vi "Basic Call Object Method.vi"(8 "Error In":errorcluster, 9 "args":string, 10 "method":string, 11 "object name":string) -> (0 "Error Out":errorcluster, 3 "concatened string":string)   [LabVIEW 2014]
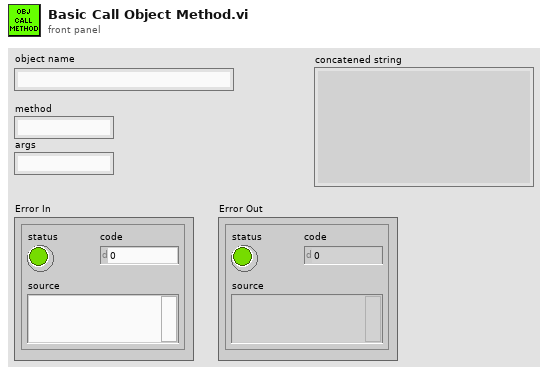
[diagram p1: front panel]
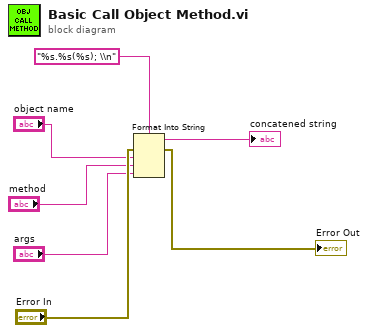
[diagram p0: block diagram]
diagram:
  n1 = Format Into String(format string="%s.%s(%s); \\n", error in="Error In", "object name", "method", "args") -> (resulting string=→"concatened string":string, error out=→"Error Out":errorcluster)  [unwired: 1 in]
